vi "App - analyze RUS V6.vi"() -> ()   [LabVIEW 2018] (continued)
              tunnel: w691 -> [_ w703]
              tunnel: w690 -> [_ w702]
              frame False {
                n263 = Initialize Array("" ("name or relative path"), 0 ("dimension size")) -> ()  [unwired: 1 out]
              }
              frame True {
                n264 = call "freq file read-write controller.vi"("Sweep folder path"=w702, "action"=save-read_action."update read list", "save/read"=w703) -> ("save/read OUT"=w701:refnum<vi>)  [unwired: 6 in, 2 out]
                n265 = call "freq file read-write controller.vi"("action"=save-read_action."lookup read number", "Numeric"=w699, "save/read"=w701) -> ("save/read OUT"=w698:refnum<vi>)  [unwired: 6 in, 2 out]
                n266 = call "freq file read-write controller.vi"("action"=save-read_action."copy read from read ring", "save/read"=w698) -> ()  [unwired: 7 in, 3 out]
              }
            }
          }
          frame "new temperature folder" {
            # "input is temperature folder path"
            # "attemp to help to not accidentally \noverwrite existing freqout file NOT FINISHED"
            n267 = call <vilib>:"Check if File or Folder Exists.vi"("path"=w715) -> ("file or folder exists?"=w723:bool, "dup path"=w722:path)  [unwired: 8 in, 1 out]
            n268 = flat-sequence {
              tunnel: w723 -> [w734]
              tunnel: w722 -> [w733]
              tunnel: [w732] -> w716
              tunnel: [w731] -> w721
              tunnel: w713 -> [w730]
              tunnel: w712 -> [w729]
              tunnel: w711 -> [w728]
              tunnel: w710 -> [w727]
              tunnel: w709 -> [w726]
              tunnel: w707 -> [w725]
              tunnel: w720 -> [w802]
              tunnel: w716 -> [w801]
              tunnel: w708 -> [w800]
              frame #0 {
                n269 = case shown="True" w734 {
                  tunnel: w733 -> [_ w754]
                  tunnel: [FALSE w743] -> w732
                  tunnel: [0 w756] -> w731
                  tunnel: w730 -> [_ w748]
                  tunnel: w729 -> [_ w747]
                  tunnel: w728 -> [_ w746]
                  tunnel: w727 -> [_ w745]
                  tunnel: w726 -> [_ w744]
                  tunnel: w725 -> [_ w739]
                  frame False {
                  }
                  frame True {
                    w750 = T40."new"  # action
                    (unwired) FALSE
                    (unwired) TRUE
                    n270 = call "file list from temperatures file V5.vi"("sweep folder path  IN"=w754, "tfolder IN"=w747, "action"=w750, "monotonic segments ON/OFF"=w745) -> ("sweep path array OUT"=w752:T26[], "tfolder OUT"=w749:T30, "OK"=w741:bool, "temperature OUT"=w751:dbl[], "power  OUT"=w738:dbl[], "Magn Field  OUT"=w737:dbl[], "timestamp OUT"=w753:dbl[])  [unwired: 17 in]
                    n271 = And(x=w741, y=FALSE) -> (x .and. y?=w742:bool)
                    n272 = property on="-- loading ..." class="Bool (strict)"("Visible"=w742) -> ()  [unwired: 2 in, 2 out]
                    n273 = property on="-- loading ..." class="Bool (strict)"("Visible"=w744) -> ()  [unwired: 2 in, 2 out]
                    n274 = Array Size(array=w753) -> (size(s)=w756:i32)
                    n275 = Greater Than 0?(x=w756) -> (x > 0?=w743:bool)
                    n276 = case shown="True" w743 {
                      selector: w743 -> [_ w783]
                      tunnel: w753 -> [_ w777]
                      tunnel: w752 -> [_ w759]
                      tunnel: w756 -> [_ w784]
                      tunnel: T27 {"temperature"=0.0, "lorentzian"={"A (VHz)"=0.0, "f (Hz)"=0.0, "G (Hz)"=0.0, "phi(rad)"=0.0, "Q"=0.0, "Norm  Ampl"=0.0, "bg (V)"=0.0+0.0i, "4corners"={"z (-pi/2)"=0.0+0.0i, "z(inf)"=0.0+0.0i, "z (pi/2)"=0.0+0.0i, "z center"=0.0+0.0i, "z(0)"=0.0+0.0i, "radius"=0.0}}, "timestamp(min)"=0.0, "timestamp"=timestamp(0 s since 1904-01-01), "Magn Field(T)"=0.0} ("temperature sweep point") -> [_ w782]
                      tunnel: w751 -> [_ w760]
                      tunnel: w749 -> [_ w775]
                      tunnel: w748 -> [_ w774]
                      tunnel: w746 -> [_ w772]
                      tunnel: w739 -> [_ w767]
                      tunnel: w738 -> [_ w765]
                      tunnel: w737 -> [_ w761]
                      frame False {
                      }
                      frame True {
                        # "set temperature to the middle of the range"
                        n277 = disable-structure shown="Enabled" {
                          disable-tunnel: w777 -> [w797 w799]
                          disable-tunnel: [w796 w799] -> w757
                          frame Enabled {
                            # "set origin to zero"
                            n278 = Array Max & Min(array=w797) -> (min value=w798:dbl)  [unwired: 3 out]
                            n279 = Subtract(x=w797, y=w798) -> (x-y=w796:dbl[])
                          }
                          frame Disabled {
                          }
                        }
                        n280 = local write "in sweep folder"(w783) -> ()
                        n281 = Initialize Array(0.0 ("element"), w784) -> (→"frequency points" →"attenuation points" →"phase points" →"Fit delta f points" →"Fit F points" →"ampl points":dbl[])
                        n282 = Initialize Array(w782, w784) -> (w762:T27[])
                        n283 = Unbundle By Name(w775) -> ("9folder path"=w776:path)
                        n284 = local write "t.folder file path array"(w759) -> ()
                        n285 = local write "tfolder"(w775) -> ()
                        n286 = local write "time points"(w757) -> ()
                        n287 = Array Size(array=w757) -> (size(s)=w787:i32)
                        n288 = local write "9w folder path"(w776) -> ()
                        n289 = Index Array(array=w757, index=0) -> ()  [unwired: 1 out]
                        n290 = Decrement(x=w787) -> (x-1=w788:i32)
                        n291 = Index Array(array=w757, index=w788) -> (element=w768:dbl)
                        n292 = call "cursor window logic V2.vi"("cursor window action"=cursor_window_action."check", "cursor window in"=w774) -> ("cursor window out"=w773:refnum<vi>)  [unwired: 8 in, 1 out]
                        n293 = Threshold 1D Array(2:w768, 3:w757) -> (0:w763:dbl)  [unwired: 1 in]
                        n294 = for {
                          tunnel: w762 -> [w795] mode=indexing
                          tunnel: [w794] -> w758 mode=indexing
                          tunnel: w761 -> [w793] mode=indexing
                          tunnel: w760 -> [w792] mode=indexing
                          tunnel: w759 -> [w791] mode=indexing
                          tunnel: w757 -> [w789] mode=indexing
                          n295 = Unbundle By Name(w791) -> ("last mod"=w790:timestamp)
                          n296 = Bundle By Name(cluster=w795, "temperature"=w792, "Magn Field(T)"=w793, "timestamp(min)"=w789, "timestamp"=w790) -> (w794:T27)
                        }
                        n297 = Index Array(array=w759, index=w763) -> (element=w781:T26)
                        n298 = Unbundle By Name(w781) -> ("temperature"=w780:dbl, "Magn Field(T)"=w764:dbl)
                        n299 = call "cursor window logic V2.vi"("cursor window action"=cursor_window_action."change center", "center"=w768, "cursor window in"=w773) -> ()  [unwired: 7 in, 2 out]
                        n300 = local write "lorentzian points"(w758) -> ()
                        n301 = local write "Magn Field points"(w761) -> ()
                        n302 = local write "temperature points"(w760) -> ()
                        n303 = local write "power points"(w765) -> ()
                        n304 = local write "temperature(K)"(w780) -> ()
                        n305 = local write "magn field(T)"(w764) -> ()
                        n306 = local write "time (min)"(w768) -> ()
                        n307 = local write "current index"(w763) -> ()
                        n308 = call "replace cursor - plot ref.vi"("action"=enum16{"", "read", "write"}."write", "cursor index"=0, "new X"=w768, "Plot ref in"=w772) -> ()  [unwired: 5 in, 3 out]
                        n309 = call "follow the peak controller.vi"("action"=follow_the_peak_action."make dirty", "follow the peak ref"=w767) -> ()  [unwired: 8 in, 2 out]
                      }
                    }
                  }
                }
              }
              frame #1 {
                n310 = case shown="True" w801 {
                  tunnel: w802 -> [_ w806]
                  tunnel: w800 -> [_ w805]
                  frame False {
                  }
                  frame True {
                    w807 = "new temperature"  # t.folder
                    n311 = Generate User Event(user event=w806, event data cluster=w807) -> (error out=w803:errorcluster)  [unwired: 2 in, 1 out]
                    n312 = Generate User Event(user event=w805, event data cluster="redraw:time" ("t.folder"), error in=w803) -> ()  [unwired: 1 in, 2 out]
                  }
                }
              }
            }
            n313 = call "freq file read-write controller.vi"("action"=save-read_action."init save file", "save/read"=w706) -> ()  [unwired: 7 in, 3 out]
            n314 = Select(t=u32 16777222, s=w716, f=u32 16719872) -> (s? t:f=w717:u32)
            n315 = property on="Sweep folder path" class="Path"("Text.TextColor"=w717) -> ()  [unwired: 2 in, 2 out]
            n316 = case shown="True" w716 {
              tunnel: T37."Enabled" ("Disabled") -> [_ w724]
              frame False {
              }
              frame True {
                n317 = property on="Tab : temperature folder" class="TabCtl (strict)"("DisabledEnum"=w724) -> ()  [unwired: 2 in, 2 out]
              }
            }
            "files in t.folder" <- w721
          }
          frame "not in temperature folder" {
            w808 = TRUE  # Visible
            w809 = T37."Disabled and Grayed Out"  # Disabled
            n318 = local write "in sweep folder"(w810) -> ()
            n319 = property on="back to temperature folder" class="Bool"("Visible"=w808) -> ()  [unwired: 2 in, 2 out]
            n320 = property on="Tab : temperature folder" class="TabCtl (strict)"("DisabledEnum"=w809) -> ()  [unwired: 2 in, 2 out]
          }
          frame "update freq/atten" {
            n321 = case shown="True" w813 {
              tunnel: w821 -> [_ w831]
              tunnel: w820 -> [_ w830]
              tunnel: w819 -> [_ w829]
              tunnel: w818 -> [_ w828]
              tunnel: w817 -> [_ w827]
              tunnel: w816 -> [_ w826]
              tunnel: w815 -> [_ w825]
              tunnel: w814 -> [_ w824]
              tunnel: w812 -> [_ w823]
              tunnel: w811 -> [_ w822]
              frame False {
              }
              frame True {
                n322 = flat-sequence {
                  tunnel: w831 -> [_]
                  tunnel: w829 -> [w868]
                  tunnel: w828 -> [w867]
                  tunnel: w827 -> [w866]
                  tunnel: w826 -> [w865]
                  tunnel: w825 -> [w864]
                  tunnel: w824 -> [w837]
                  tunnel: w823 -> [w836]
                  tunnel: w822 -> [w834]
                  tunnel: w830 -> [w875]
                  frame #0 {
                    w841 = enum16{"", "read", "write"}."write"  # action
                    w845 = enum16{"", "read", "write"}."write"  # action
                    n323 = local read "time (min)"() -> (w854:dbl)
                    n324 = Threshold 1D Array(2:w854, 3:w867) -> (0:w833:dbl)  [unwired: 1 in]
                    n325 = Index Array(array=w866, index=w833) -> (element=w847:dbl)
                    n326 = Index Array(array=w834, index=w833) -> (element=w832:dbl)
                    n327 = local read "attenuation points"() -> (w859:dbl[])
                    n328 = local read "frequency points"() -> (w860:dbl[])
                    n329 = call "freq file read-write controller.vi"("action"=save-read_action."saved file dirty", "save/read"=w836) -> ()  [unwired: 7 in, 3 out]
                    n330 = in-place {
                      in-place-border: w868 -> [w871]
                      in-place-border: w847 -> [w870]
                      in-place-border: w832 -> [w869]
                      n331 = in-place-array #1(w865, w833) -> (w873:T27)
                      n332 = Bundle By Name(cluster=w873, "lorentzian"=w871, "temperature"=w870, "Magn Field(T)"=w869) -> (w872:T27)
                      n333 = in-place-array #1(w872) -> (w855:T27[])  [unwired: 1 out]
                    }
                    n334 = Unbundle By Name(w868) -> ("A (VHz)"=w853:dbl, "phi(rad)"=w857:dbl, "G (Hz)"=w861:dbl, "f (Hz)"=w843:dbl)
                    n335 = local read "phase points"() -> (w858:dbl[])
                    n336 = local read "ampl points"() -> (w852:dbl[])
                    n337 = Replace Array Subset(array=w858, new element=w857, index=w833) -> (w856:dbl[])
                    n338 = Replace Array Subset(array=w852, new element=w853, index=w833) -> (w851:dbl[])
                    n339 = Replace Array Subset(array=w859, new element=w861, index=w833) -> (w862:dbl[])
                    n340 = Replace Array Subset(array=w860, new element=w843, index=w833) -> (w863:dbl[])
                    n341 = Build Array(w847) -> (w848:dbl[])
                    n342 = local write "lorentzian points"(w855) -> ()
                    n343 = local write "phase points"(w856) -> ()
                    n344 = local write "frequency points"(w863) -> ()
                    n345 = local write "attenuation points"(w862) -> ()
                    n346 = local write "ampl points"(w851) -> ()
                    n347 = call "fit function selector.vi"("fit using"=w837, "temperature"=w848, "best fit parameters"=w864) -> ("freq out"=w849:dbl[])  [unwired: 6 in, 2 out]
                    n348 = Index Array(array=w849, index=0 ("cursor index")) -> (element=w842:dbl)
                    n349 = Subtract(x=w843, y=w842) -> (x-y=w839:dbl)
                    n350 = control-ref of="Plot: frequency vs T"() -> (w846:refnum<vi>)
                    n351 = call "replace cursor - plot ref.vi"("action"=w845, "cursor index"=1, "new  Y"=w843, "Plot ref in"=w846) -> ()  [unwired: 5 in, 3 out]
                    n352 = control-ref of="Plot: delta f"() -> (w838:refnum<vi>)
                    n353 = call "replace cursor - plot ref.vi"("action"=w841, "cursor index"=1, "new  Y"=w839, "Plot ref in"=w838) -> ()  [unwired: 5 in, 3 out]
                  }
                  frame #1 {
                    w874 = "calculation finished"  # talk to the first loop
                    n354 = Generate User Event(user event=w875, event data cluster=w874) -> ()  [unwired: 2 in, 2 out]
                  }
                }
              }
            }
          }
          frame "clear freq points" {
            n355 = case shown="True" w877 {
              tunnel: w879 -> [_ w884]
              tunnel: w878 -> [_ w883]
              tunnel: w876 -> [_ w880]
              frame False {
              }
              frame True {
                n356 = local read "attenuation points"() -> (w896:dbl[])
                n357 = local read "frequency points"() -> (w897:dbl[])
                n358 = local read "Fit delta f points"() -> (w890:dbl[])
                n359 = local read "phase points"() -> (w886:dbl[])
                n360 = local read "ampl points"() -> (w882:dbl[])
                n361 = local read "Fit F points"() -> (w889:dbl[])
                n362 = Unbundle By Name(T27 {"temperature"=0.0, "lorentzian"={"A (VHz)"=0.0, "f (Hz)"=0.0, "G (Hz)"=0.0, "phi(rad)"=0.0, "Q"=0.0, "Norm  Ampl"=0.0, "bg (V)"=0.0+0.0i, "4corners"={"z (-pi/2)"=0.0+0.0i, "z(inf)"=0.0+0.0i, "z (pi/2)"=0.0+0.0i, "z center"=0.0+0.0i, "z(0)"=0.0+0.0i, "radius"=0.0}}, "timestamp(min)"=0.0, "timestamp"=timestamp(0 s since 1904-01-01), "Magn Field(T)"=0.0} ("temperature sweep point")) -> ("lorentzian"=w894:T11)
                n363 = for {
                  shift-right: [w913] -> w892
                  shift-left: w896 -> [w915]
                  shift-right: [w906] -> w893
                  shift-left: w883 -> [w903]
                  shift-right: [w914] -> w891
                  shift-left: w897 -> [w916]
                  tunnel: w884 -> [w904] mode=indexing
                  tunnel: w894 -> [w905]
                  shift-right: [w912] -> w888
                  shift-left: w890 -> [w909]
                  shift-right: [w911] -> w887
                  shift-left: w889 -> [w910]
                  shift-right: [w907] -> w885
                  shift-left: w886 -> [w908]
                  shift-right: [w899] -> w881
                  shift-left: w882 -> [w900]
                  tunnel: w880 -> [w898] mode=indexing
                  i -> [w902]
                  w901 = 0.0 ("new element/subarray")
                  n364 = in-place {
                    in-place-border: w905 -> [w921]
                    in-place-border: w904 -> [w920]
                    in-place-border: w898 -> [w917]
                    n365 = in-place-array #2(w903, w902) -> (w918:T27)
                    n366 = Bundle By Name(cluster=w918, "Magn Field(T)"=w917, "temperature"=w920, "lorentzian"=w921) -> (w919:T27)
                    n367 = in-place-array #2(w919) -> (w906:T27[])  [unwired: 1 out]
                  }
                  n368 = Replace Array Subset(array=w916, new element=w901, index=w902) -> (w914:dbl[])
                  n369 = Replace Array Subset(array=w909, new element=w901, index=w902) -> (w912:dbl[])
                  n370 = Replace Array Subset(array=w910, new element=w901, index=w902) -> (w911:dbl[])
                  n371 = Replace Array Subset(array=w900, new element=w901, index=w902) -> (w899:dbl[])
                  n372 = Replace Array Subset(array=w908, new element=w901, index=w902) -> (w907:dbl[])
                  n373 = Replace Array Subset(array=w915, new element=w901, index=w902) -> (w913:dbl[])
                }
                n374 = local write "lorentzian points"(w893) -> ()
                n375 = local write "frequency points"(w891) -> ()
                n376 = local write "attenuation points"(w892) -> ()
                n377 = local write "phase points"(w885) -> ()
                n378 = local write "Fit delta f points"(w888) -> ()
                n379 = local write "Fit F points"(w887) -> ()
                n380 = local write "ampl points"(w881) -> ()
              }
            }
          }
          frame "new temperature" {
            n381 = case shown="True" w923 {
              tunnel: w930 -> [_ w941]
              tunnel: w923 -> [_ w940]
              tunnel: w929 -> [_ w939]
              tunnel: w928 -> [_ w938]
              tunnel: w927 -> [_ w937]
              tunnel: w926 -> [_ w936]
              tunnel: w925 -> [_ w935]
              tunnel: w924 -> [_ w934]
              tunnel: w922 -> [_ w931]
              frame False {
              }
              frame True {
                # "calculation  for the next temperature uses the two cursor brackets that are set here"
                # "logic : this and othe othe events are chaned:\n any of them induce the down stream events to execute"
                n382 = flat-sequence {
                  tunnel: w940 -> [w967]
                  tunnel: w939 -> [w964]
                  tunnel: w938 -> [w956]
                  tunnel: w937 -> [w957]
                  tunnel: w936 -> [w963]
                  tunnel: w935 -> [w962]
                  tunnel: [w961] -> w943
                  tunnel: [w960] -> w942
                  tunnel: w931 -> [w948]
                  tunnel: w934 -> [w988]
                  tunnel: w943 -> [w987]
                  tunnel: w942 -> [w979]
                  tunnel: w933 -> [w982]
                  tunnel: w932 -> [w980]
                  tunnel: w941 -> [w990]
                  frame #0 {
                    n383 = Unbundle By Name(w962) -> ("G (Hz)"=w953:dbl, "f (Hz)"=w958:dbl)
                    n384 = call "follow the peak controller.vi"("action"=follow_the_peak_action."check", "follow the peak ref"=w948) -> ("follow the peak OUT"=w945:T7)  [unwired: 8 in, 1 out]
                    n385 = local read "time (min)"() -> (w961:dbl)
                    n386 = Unbundle By Name(w945) -> ("omega ?"=w947:bool)
                    n387 = Threshold 1D Array(2:w961, 3:w963) -> (0:w966:dbl)  [unwired: 1 in]
                    n388 = Compound Arithmetic op=AND(w967, w947) -> (w954:bool)
                    n389 = case shown="True" w954 {
                      tunnel: w958 -> [_ w977]
                      tunnel: w957 -> [_ w976]
                      tunnel: w956 -> [_ w975]
                      tunnel: [w968 FALSE] -> _
                      tunnel: [w968 w973] -> w955
                      tunnel: w953 -> [_ w971]
                      tunnel: w945 -> [_ w969]
                      frame False {
                        w968 = FALSE
                      }
                      frame True {
                        n390 = call "follow the peak.vi"("omega(0)"=w977, "gamma"=w971, "follow the peak Con"=w969, "cursor bracket - data 2"=w975, "cursor bracket - fragment 2"=w976) -> ("interpolated omega"=→"interpolated omega":dbl, "interpolated gamma"=→"interpolated gamma":dbl, "follow the peak is clean out"=w973:bool)  [unwired: 8 in]
                      }
                    }
                    n391 = Index Array(array=w964, index=w966) -> (element=w965:T26)
                    n392 = Unbundle By Name(w965) -> ("temperature"=w960:dbl, "file path"=w959:path, "Magn Field(T)"=w944:dbl)
                    n393 = Compound Arithmetic op=AND(w955, w954) -> (w952:bool)
                    n394 = Select(t=follow_the_peak_action."make clean" ("action"), s=w952, f=follow_the_peak_action."make clean" ("action")) -> (s? t:f=w949:T33)
                    n395 = local write "temperature(K)"(w960) -> ()
                    n396 = local write "magn field(T)"(w944) -> ()
                    n397 = local write "file path"(w959) -> ()
                    n398 = call "follow the peak controller.vi"("action"=w949, "follow the peak ref"=w948) -> ()  [unwired: 8 in, 2 out]
                  }
                  frame #1 {
                    w981 = enum16{"", "read", "write"}."write"  # action
                    w984 = enum16{"", "read", "write"}."write"  # action
                    w986 = enum16{"", "read", "write"}."write"  # action
                    n399 = call "replace cursor - plot ref.vi"("action"=w984, "cursor index"=1, "new X"=w979, "Plot ref in"=w982) -> ()  [unwired: 5 in, 3 out]
                    n400 = call "replace cursor - plot ref.vi"("action"=w981, "cursor index"=1, "new X"=w979, "Plot ref in"=w980) -> ()  [unwired: 5 in, 3 out]
                    n401 = call "replace cursor - plot ref.vi"("action"=w986, "cursor index"=5, "new  Y"=w979, "new X"=w987, "Plot ref in"=w988) -> ()  [unwired: 4 in, 3 out]
                  }
                  frame #2 {
                    # "send \"new file\" event"
                    n402 = Generate User Event(user event=w990, event data cluster="calc:new file" ("event data")) -> ()  [unwired: 2 in, 2 out]
                  }
                }
                n403 = control-ref of="Plot: frequency vs T"() -> (w933:refnum<vi>)
                n404 = control-ref of="Plot: delta f"() -> (w932:refnum<vi>)
              }
            }
          }
          frame "set time to left" {
            # "cursor bracket -- bounds"
            n405 = call "cursor window logic V2.vi"("cursor window action"=cursor_window_action."check", "cursor window in"=w1002) -> ("cursor window out"=w1001:T24)  [unwired: 8 in, 1 out]
            n406 = Unbundle By Name(w1001) -> ("left"=w1000:dbl)
            n407 = Threshold 1D Array(2:w1000, 3:w998) -> (0:w992:dbl)  [unwired: 1 in]
            n408 = Index Array(array=w999, index=w992) -> (element=w996:dbl)
            n409 = Index Array(array=w993, index=w992) -> (element=w991:dbl)
            n410 = Index Array(array=w998, index=w992) -> (element=w997:dbl)
            n411 = local write "temperature(K)"(w996) -> ()
            n412 = local write "magn field(T)"(w991) -> ()
            n413 = local write "time (min)"(w997) -> ()
            n414 = Generate User Event(user event=w994, event data cluster="new temperature" ("event data")) -> ()  [unwired: 2 in, 2 out]
          }
          frame "follow the peak -- init" {
            n415 = call "follow the peak controller.vi"("action"=follow_the_peak_action."make dirty", "follow the peak ref"=w1005) -> ()  [unwired: 8 in, 2 out]
          }
          frame "next peak" {
            # "\";\""
            n416 = Unbundle By Name(w1012) -> ("f (Hz)"=w1007:dbl)
            n417 = call "freq file read-write controller.vi"("action"=save-read_action."nearest right", "Numeric"=w1007, "save/read"=w1009) -> ("Numeric out"=w1006:dbl)  [unwired: 6 in, 2 out]
            n418 = call "Q - not nan and gtr than zero.vi"("Numeric"=w1006) -> ("Boolean"=w1013:bool)  [unwired: 10 in]
            n419 = case shown="True" w1013 {
              tunnel: w1011 -> [_ w1016]
              tunnel: w1006 -> [_ w1015]
              tunnel: w1010 -> [_ w1014]
              frame False {
              }
              frame True {
                n420 = flat-sequence {
                  tunnel: w1016 -> [w1019]
                  tunnel: w1015 -> [w1018]
                  tunnel: w1014 -> [w1020]
                  frame #0 {
                    n421 = call "cursor window logic V2.vi"("cursor window action"=cursor_window_action."change center", "center"=w1018, "cursor window in"=w1019) -> ()  [unwired: 7 in, 2 out]
                  }
                  frame #1 {
                    w1021 = "calc:new cursor bracket"  # event data
                    n422 = Generate User Event(user event=w1020, event data cluster=w1021) -> ()  [unwired: 2 in, 2 out]
                  }
                }
              }
            }
          }
          frame "increment peak index" {
            # ":"
            n423 = call "freq file read-write controller.vi"("action"=save-read_action."increment read from", "save/read"=w1023) -> ()  [unwired: 7 in, 3 out]
          }
          frame "latest temperature" {
            w1034 = enum16{"hide", "show x", "show y", "show (x,y)"}."hide"  # label
            w1035 = enum16{"", "read", "write"}."write"  # action
            w1036 = "same"  # next temperature
            n424 = Array Size(array=w1033) -> (size(s)=w1037:i32)
            n425 = Decrement(x=w1037) -> (x-1=w1025:i32)
            n426 = Index Array(array=w1032, index=w1025) -> (element=w1031:dbl)
            n427 = Index Array(array=w1026, index=w1025) -> (element=w1024:dbl)
            n428 = Index Array(array=w1033, index=w1025) -> (element=w1027:dbl)
            n429 = local write "magn field(T)"(w1024) -> ()
            n430 = local write "time (min)"(w1027) -> ()
            n431 = local write "temperature(K)"(w1031) -> ()
            n432 = call "replace cursor - plot ref.vi"("label"=w1034, "action"=w1035, "cursor index"=0, "new X"=w1027, "Plot ref in"=w1029) -> ()  [unwired: 4 in, 3 out]
            n433 = Generate User Event(user event=w1028, event data cluster=w1036) -> ()  [unwired: 2 in, 2 out]
          }
        }
      }
      event "Sweep folder path": Value Change; "Sweep folder path": Mouse Down {
        n434 = event-data() -> ()  [unwired: 1 in, 1 out]
        n435 = flat-sequence {
          tunnel: w1040 -> [w1043]
          tunnel: [w1042] -> w1039
          tunnel: [w1045] -> _
          tunnel: w1039 -> [w1046]
          tunnel: w1038 -> [w1047]
          frame #0 {
            w1044 = "new temperature folder"  # t.folder
            n436 = Generate User Event(user event=w1043, event data cluster=w1044) -> (error out=w1042:errorcluster)  [unwired: 2 in, 1 out]
          }
          frame #1 {
            n437 = Generate User Event(user event=w1047, event data cluster="redraw:time", error in=w1046) -> (error out=w1045:errorcluster)  [unwired: 1 in, 1 out]
          }
        }
      }
      event "back to temperature folder": Value Change {
        w1049 = FALSE  # Visible
        w1050 = T37."Enabled"  # Disabled
        n438 = event-data() -> ()  [unwired: 1 in, 2 out]
        n439 = property on="Tab : temperature folder" class="TabCtl (strict)"("DisabledEnum"=w1050) -> ()  [unwired: 2 in, 2 out]
        n440 = property on="back to temperature folder" class="Bool"("Visible"=w1049) -> ()  [unwired: 2 in, 2 out]
      }
      event Value Change {
        w1057 = "update delta freq"  # t.folder
        w1060 = "read freq file"  # t.folder
        n441 = event-data() -> ()  [unwired: 1 in, 1 out]
        n442 = case shown="False" w1054 {
          tunnel: w1059 -> [w1061 w1063]
          tunnel: [w1061 w1062] -> w1058
          frame False {
          }
          frame True {
            w1064 = "clear freq points"  # t.folder
            n443 = Generate User Event(user event=w1063, event data cluster=w1064) -> (user event out=w1062:refnum<user-event>)  [unwired: 2 in, 1 out]
          }
        }
        n444 = call "freq file read-write controller.vi"("action"=save-read_action."read event", "save/read"=w1053) -> ()  [unwired: 7 in, 3 out]
        n445 = Generate User Event(user event=w1058, event data cluster=w1060) -> (user event out=w1055:refnum<user-event>, error out=w1056:errorcluster)  [unwired: 2 in]
        n446 = Generate User Event(user event=w1055, event data cluster=w1057, error in=w1056) -> ()  [unwired: 1 in, 2 out]
      }
      event Value Change {
        w1067 = "clear freq points"  # t.folder
        n447 = event-data() -> ()  [unwired: 1 in, 1 out]
        n448 = call "freq file read-write controller.vi"("action"=save-read_action."erase event", "save/read"=w1065) -> ()  [unwired: 7 in, 3 out]
        n449 = Generate User Event(user event=w1068, event data cluster=w1067) -> ()  [unwired: 2 in, 2 out]
      }
      event Value Change {
        w1071 = "write freq file"  # t.folder
        n450 = event-data() -> ()  [unwired: 1 in, 1 out]
        n451 = call "freq file read-write controller.vi"("action"=save-read_action."read event", "save/read"=w1069) -> ()  [unwired: 7 in, 3 out]
        n452 = Generate User Event(user event=w1072, event data cluster=w1071) -> ()  [unwired: 2 in, 2 out]
      }
      event Value Change; Mouse Enter {
        n453 = event-data() -> ()  [unwired: 1 in, 3 out]
      }
      event "file path": Value Change; "file path": Mouse Down {
        w1080 = "not in temperature folder"  # t.folder
        n454 = event-data() -> ()  [unwired: 1 in, 1 out]
        n455 = local read "file path"() -> (w1073:path)
        n456 = call <vilib>:"Check if File or Folder Exists.vi"("path"=w1073) -> ("file or folder exists?"=w1075:bool)  [unwired: 8 in, 2 out]
        n457 = Generate User Event(user event=w1081, event data cluster=w1080) -> (error out=w1079:errorcluster)  [unwired: 2 in, 1 out]
        n458 = Select(t=u32 16777222, s=w1075, f=u32 16719872) -> (s? t:f=w1076:u32)
        n459 = property on="file path" class="Path"("Text.TextColor"=w1076) -> ()  [unwired: 2 in, 2 out]
        n460 = case shown="True" w1075 {
          tunnel: w1074 -> [_ w1084]
          tunnel: w1079 -> [_ w1083]
          frame False {
          }
          frame True {
            w1082 = "calc:new file"  # calc
            n461 = Generate User Event(user event=w1084, event data cluster=w1082, error in=w1083) -> ()  [unwired: 1 in, 2 out]
          }
        }
      }
      event Timeout {
        n462 = event-data() -> ()  [unwired: 1 in, 2 out]
      }
    }
  }
  n463 = Create User Event(user event datatype=w30) -> (user event=w43:refnum<user-event>)  [unwired: 1 in, 1 out]
  n464 = Create User Event(user event datatype=w46) -> (user event=w45:refnum<user-event>)  [unwired: 1 in, 1 out]
  n465 = Create User Event(user event datatype=w40) -> (user event=w39:refnum<user-event>)  [unwired: 1 in, 1 out]
  n466 = Create User Event(user event datatype=w31) -> (user event=w27:refnum<user-event>)  [unwired: 1 in, 1 out]
  n467 = Create User Event(user event datatype=w38) -> (user event=w37:refnum<user-event>)  [unwired: 1 in, 1 out]
  n468 = call "cursor window - init all.vi"("cursor bracket:  Time 2"=w22, "cursor bracket: fragment 2"=w25, "cursor bracket:  All, zoom 2"=w23, "cursor bracket:  All, data window 2"=w24, "Plot: Time"=w21, "Plot:  Fragment"=w26, "cursor bracket:  All, show 2"=w19, "Plot: All"=w20) -> ()
  n469 = control-ref of="slide control"() -> (w4:refnum<vi>)
  n470 = register-events(w17, w44, w43, w45, w39, w27, w37, w33) -> (reference out=w49:refnum<event-registration>)  [unwired: 2 in, 1 out]
  n471 = call "slide controller.vi"("slide action"=slide_action."init", "slide control"=w4) -> ("slide control OUT"=w3:refnum<vi>)  [unwired: 6 in, 3 out]
  n472 = while {
    tunnel: w49 -> [w1133]
    tunnel: w16 -> [w1132]
    tunnel: w17 -> [w1131]
    tunnel: w44 -> [w1129]
    tunnel: w45 -> [w1127]
    tunnel: w43 -> [w1126]
    tunnel: w39 -> [w1125]
    tunnel: w27 -> [w1124]
    tunnel: w18 -> [w1123]
    tunnel: w37 -> [w1122]
    tunnel: w28 -> [_]
    tunnel: w20 -> [_]
    tunnel: w3 -> [_]
    i -> [w1093]
    stop <- FALSE ("Boolean") stop-if-true
    n473 = local read "cursor bracket: All, data window"() -> (w1103:T24)
    n474 = local read "parameters: center detection"() -> (w1116:T21)
    n475 = Wait (ms)(milliseconds to wait=u32 3) -> ()  [unwired: 1 out]
    n476 = Equal To 0?(x=w1093) -> (x = 0?=w1092:bool)
    n477 = local read "parameters: wavepacket"() -> (w1113:T16)
    n478 = local read "cursor bracket: fragment"() -> (w1104:T24)
    n479 = local read "parameters: omega map"() -> (w1115:T22)
    n480 = control-ref of="save/read"() -> (w1089:refnum<vi>)
    n481 = local read "plot scale: Geometry"() -> (w1121:T28)
    n482 = local read "cursor bracket: Time"() -> (w1101:T24)
    n483 = local read "Sweep folder path"() -> (w1112:path)
    n484 = local read "in sweep folder"() -> (w1118:bool)
    n485 = local read "complex region"() -> (w1114:T25)
    n486 = local read "9w folder path"() -> (w1111:path)
    n487 = control-ref of="follow the peak"() -> (w1091:refnum<vi>)
    n488 = local read "lorentzian"() -> (w1117:T11)
    n489 = control-ref of="Plot: All"() -> (w1102:refnum<vi>)
    n490 = control-ref of="Plot: complex plane"() -> (w1105:refnum<vi>)
    n491 = control-ref of="Plot: fragment"() -> (w1106:refnum<vi>)
    n492 = control-ref of="Plot: Time"() -> (w1100:refnum<vi>)
    n493 = control-ref of="slide control"() -> (w1090:refnum<vi>)
    n494 = local read "section"() -> (w1119:i32)
    n495 = local read "tfolder"() -> (w1120:T30)
    n496 = control-ref of="cursor bracket: All, data window"() -> (w1108:refnum<vi>)
    n497 = control-ref of="cursor bracket: All,  zoom"() -> (w1109:refnum<vi>)
    n498 = control-ref of="cursor bracket: fragment"() -> (w1107:refnum<vi>)
    n499 = control-ref of="cursor bracket: Time"() -> (w1110:refnum<vi>)
    n500 = control-ref of="Plot: frequency vs H"() -> (w1086:refnum<vi>)
    n501 = control-ref of="Plot: attenuation vs H"() -> (w1085:refnum<vi>)
    n502 = control-ref of="Plot: gamma vs power"() -> (w1087:refnum<vi>)
    n503 = control-ref of="Plot: frequency vs power"() -> (w1088:refnum<vi>)
    n504 = control-ref of="Plot: Time"() -> (w1094:refnum<vi>)
    n505 = control-ref of="Plot: frequency vs T"() -> (w1097:refnum<vi>)
    n506 = control-ref of="Plot: attenuation vs T"() -> (w1098:refnum<vi>)
    n507 = control-ref of="Plot: df/dT"() -> (w1099:refnum<vi>)
    n508 = control-ref of="Plot: delta f"() -> (w1096:refnum<vi>)
    n509 = event shown="[18] <redraw>: User Event" {
      selector: w1133 -> [_ _ _ _ _ _ _ _ _ _ _ _ _ _ _ _ _ _ _ _ _ _ _ _ _ _ _ _ _ _ _ _ _ _ _ _ _ _ _ _ _ _ _ _ _]
      dyn-events: _ -> [_ _ _ _ _ _ _ _ _ _ _ _ _ _ _ _ _ _ _ _ _ _ _ _ _ _ _ _ _ _ _ _ _ _ _ _ _ _ _ _ _ _ _ _ _]
      timeout: _ -> [_ _ _ _ _ _ _ _ _ _ _ _ _ _ _ _ _ _ _ _ _ _ _ _ _ _ _ _ _ _ _ _ _ _ _ _ _ _ _ _ _ _ _ _ _]
      tunnel: w1132 -> [_ _ w1213 _ _ _ _ w1577 _ _ _ _ _ _ _ _ _ _ _ _ _ _ _ _ _ _ _ _ _ _ _ _ _ _ _ _ _ _ _ _ _ _ w2370 w2385 w2415]
      tunnel: w1131 -> [w1142 _ w1221 _ _ _ _ w1576 _ _ _ _ _ _ _ w1664 _ _ w1827 _ _ _ _ _ _ _ _ _ _ _ _ _ _ _ w2284 _ _ _ _ _ w2364 w2367 _ _ _]
      tunnel: [_ _ _ _ _ _ _ _ _ _ _ _ _ _ _ _ _ _ _ _ _ _ _ _ _ _ _ _ _ _ _ _ _ _ _ "help (h)" _ _ _ _ "plot filter progress?" _ _ _ _] -> _
      tunnel: [_ _ _ _ _ w1555 _ _ _ _ _ _ _ _ _ _ _ _ _ _ _ _ _ _ _ _ _ _ _ _ _ _ _ _ _ "help toggle" _ _ _ _ _ _ _ _ _] -> _
      tunnel: FALSE ("Boolean") -> [_ _ _ _ _ w1555 w1562 _ _ _ _ _ _ _ _ _ _ _ _ _ _ _ _ _ _ _ _ _ _ _ _ _ _ _ _ _ _ _ _ _ _ _ w2369 _ _]
      tunnel: w1129 -> [_ w1203 w1222 _ _ w1557 w1565 _ _ _ _ w1611 _ _ _ w1665 _ _ _ _ _ _ _ _ _ _ _ _ _ _ _ _ _ _ _ _ _ _ _ _ _ _ _ _ _]
      tunnel: TRUE ("Boolean") -> [_ _ _ _ _ w1556 _ _ _ _ _ _ _ _ _ _ _ _ _ _ _ _ _ _ _ _ _ _ _ _ _ _ _ _ _ _ _ _ _ _ _ _ _ _ _]
      tunnel: [_ _ _ _ _ _ w1563 _ w1599 w1603 w1606 w1609 _ _ _ _ _ _ _ _ _ _ _ _ _ _ _ _ _ _ _ _ _ _ _ _ _ _ _ _ _ _ _ _ _] -> _
      tunnel: [_ _ _ _ _ _ _ _ _ "c.plane scale" _ _ _ _ _ _ _ _ _ _ _ _ _ _ _ _ _ _ _ _ _ _ _ _ _ _ _ _ _ _ _ _ _ _ _] -> _
      tunnel: w1127 -> [_ _ w1220 _ _ _ _ _ _ _ _ _ _ _ _ _ _ _ _ _ _ _ _ _ _ _ _ _ _ _ _ _ _ _ _ _ _ _ _ _ _ _ _ _ _]
      tunnel: [_ _ _ _ _ _ _ _ _ _ "show all cursors (c)" _ _ _ _ _ _ _ _ _ _ _ _ _ _ _ _ _ _ _ _ _ _ _ _ _ _ _ _ _ _ _ _ _ _] -> _
      tunnel: w1126 -> [_ _ w1215 _ _ _ _ w1572 _ _ w1607 _ _ _ _ _ _ _ _ _ _ _ _ _ _ _ _ _ _ _ _ _ _ _ _ _ _ _ _ _ _ _ _ _ _]
      tunnel: [_ _ _ _ _ _ w1562 _ _ _ _ _ "show all pallets (p)" _ _ _ _ _ _ _ _ _ _ _ _ _ _ _ _ _ _ _ _ _ _ _ _ _ _ _ _ _ _ _ _] -> _
      tunnel: w1125 -> [_ _ w1219 _ _ _ _ _ _ _ _ _ w1614 _ _ _ _ _ _ _ _ _ _ _ _ _ _ _ _ _ _ _ _ _ _ _ _ _ _ _ _ _ _ _ _]
      tunnel: [_ _ _ _ _ _ _ w1571 _ _ _ _ w1612 _ _ _ _ _ _ _ _ _ _ _ _ _ _ _ _ _ _ _ _ _ _ _ _ _ _ _ _ _ _ _ _] -> _
      tunnel: w1124 -> [_ _ w1218 _ _ _ _ w1573 _ w1602 _ _ _ _ _ w1663 _ _ w1797 _ w2141 _ _ _ _ _ _ _ _ _ _ _ _ _ _ _ _ _ _ _ _ _ _ _ _]
      tunnel: w1123 -> [w1141 _ w1217 w1432 w1486 _ _ w1575 _ _ _ _ _ _ _ _ _ _ _ _ _ _ w2160 _ _ _ _ _ _ _ _ _ _ _ _ _ _ _ _ _ _ _ _ _ _]
      tunnel: w1122 -> [_ _ w1216 _ _ _ _ _ _ _ _ _ _ _ _ _ _ _ _ _ _ _ _ _ _ _ _ _ _ _ _ _ _ _ _ _ _ _ _ _ _ _ _ _ _]
      tunnel: w1121 -> [_ _ _ _ _ _ _ _ _ _ _ _ _ _ _ _ _ _ _ _ _ _ _ _ _ _ _ _ _ _ _ _ _ _ _ _ _ _ _ _ _ _ _ _ _]
      tunnel: [_ _ _ _ _ _ _ _ _ _ _ _ _ _ _ _ _ _ _ _ _ _ _ _ _ _ _ _ _ _ w2250 _ _ _ _ _ _ _ _ _ _ _ _ _ _] -> _
      tunnel: w1120 -> [_ _ _ _ _ _ _ _ _ _ _ _ _ _ _ _ _ _ w1817 _ _ _ _ _ _ _ _ _ _ _ _ _ _ w2276 w2287 _ _ _ _ _ _ _ _ _ _]
      tunnel: w1119 -> [_ _ _ _ _ _ _ _ _ _ _ _ _ _ _ _ _ _ _ _ _ _ _ _ _ _ _ _ _ _ _ _ _ _ w2286 _ _ _ _ _ _ _ _ _ _]
      tunnel: w1118 -> [_ _ w1209 _ w1481 _ _ _ _ _ _ _ _ _ _ _ _ _ w1814 _ _ _ _ _ _ _ _ _ _ _ _ _ _ _ _ _ _ _ _ _ _ _ _ _ _]
      tunnel: w1117 -> [_ _ w1210 w1430 _ _ _ _ _ _ _ _ _ _ _ w1662 w1715 _ w1819 _ _ _ w2162 _ w2184 _ _ _ w2232 w2241 _ _ _ _ _ _ _ _ _ _ _ _ _ _ _]
      tunnel: w1116 -> [w1140 _ _ w1428 _ _ _ _ _ _ _ _ _ _ _ _ w1714 _ w1818 _ _ _ _ _ _ _ _ _ _ _ _ _ _ _ _ _ _ _ _ _ _ _ _ _ _]
      tunnel: w1115 -> [_ _ _ w1429 _ _ _ _ _ _ _ _ _ _ _ _ _ _ w1816 _ _ _ _ _ _ _ _ _ _ _ _ _ _ _ _ _ _ _ _ _ _ _ _ _ _]
      tunnel: w1114 -> [_ _ _ _ _ _ _ _ _ _ _ _ _ _ _ _ w1713 _ w1813 _ _ _ _ _ _ _ _ _ _ _ _ _ _ _ _ _ _ _ _ _ _ _ _ _ _]
      tunnel: w1113 -> [_ _ _ _ _ _ _ _ _ _ _ _ _ _ _ _ _ _ w1815 _ _ _ _ _ _ _ _ _ _ _ _ _ _ _ _ _ _ _ _ _ _ _ _ _ _]
      tunnel: w1112 -> [_ _ w1207 _ _ _ _ _ _ _ _ _ _ _ _ _ _ _ _ _ _ _ _ _ _ _ _ _ _ _ _ _ _ _ _ _ _ _ _ _ _ _ _ _ _]
      tunnel: w1111 -> [_ _ _ _ _ _ _ _ _ _ _ _ _ _ _ _ _ _ _ _ _ _ w2164 _ _ _ _ _ _ _ _ _ _ _ _ _ _ _ _ _ _ _ _ _ _]
      tunnel: w1110 -> [_ _ _ _ _ _ _ _ _ _ _ _ _ _ _ _ _ _ _ _ _ w2144 _ _ _ _ _ _ _ _ _ _ _ _ _ _ _ _ _ _ _ _ _ _ _]
      tunnel: w1109 -> [_ _ w1214 _ _ _ _ w1568 _ _ _ _ _ _ w1649 _ w1711 _ _ w2080 _ _ _ _ _ _ _ _ _ _ _ _ _ _ _ _ _ _ _ _ _ _ _ _ _]
      tunnel: w1108 -> [_ _ w1211 _ _ _ _ _ _ _ _ _ _ _ w1648 _ _ _ _ w2081 _ _ _ _ _ _ _ _ _ _ _ _ _ _ _ _ _ _ _ _ _ _ _ _ _]
      tunnel: w1107 -> [w1139 _ _ _ _ _ _ _ _ _ _ _ _ _ _ _ _ _ _ w2082 _ _ _ _ _ _ _ _ _ _ _ _ _ _ _ _ _ _ _ _ _ _ _ _ _]
      tunnel: w1106 -> [w1137 _ _ _ _ _ _ _ _ _ _ _ _ _ _ w1661 _ _ w1801 w2078 _ _ _ _ _ _ _ _ _ _ _ _ _ _ _ _ _ _ _ _ _ _ _ _ _]
      tunnel: w1105 -> [w1136 _ _ w1427 _ _ _ _ _ _ _ _ _ _ _ _ _ _ _ _ _ _ _ _ _ _ _ _ _ _ _ _ _ _ _ _ _ _ _ _ _ _ _ _ _]
      tunnel: w1104 -> [_ _ _ w1426 _ _ _ _ _ _ _ _ _ _ _ _ _ _ _ _ _ _ _ _ _ _ _ _ _ _ _ _ _ _ _ _ _ _ _ _ _ _ _ _ _]
      tunnel: w1103 -> [_ _ _ _ _ _ _ _ _ _ _ _ _ _ _ _ w1712 _ _ _ _ _ _ _ w2183 _ _ _ _ _ _ _ _ _ _ _ _ _ _ _ _ _ _ _ _]
      tunnel: w1102 -> [w1138 _ _ _ _ _ _ _ _ _ _ _ _ _ _ _ _ _ _ w2079 _ _ _ _ _ _ _ _ _ _ _ _ _ _ _ _ _ _ _ _ _ _ _ _ _]
      tunnel: w1101 -> [_ _ _ _ w1485 _ _ _ _ _ _ _ _ _ _ _ _ _ w1803 _ _ _ _ _ _ _ _ _ _ _ _ _ _ _ _ _ _ _ _ _ _ _ _ _ _]
      tunnel: w1100 -> [_ w1199 _ _ _ _ _ _ _ _ _ _ _ _ _ _ _ _ _ _ _ w2143 _ _ _ _ _ _ _ _ _ _ _ _ _ _ _ _ _ _ _ _ _ _ _]
      tunnel: w1099 -> [_ _ _ _ _ _ _ _ _ _ _ _ _ _ _ _ _ _ w1810 _ _ _ _ _ _ _ _ _ _ _ _ _ _ _ _ _ _ w2312 _ _ _ _ _ _ _]
      tunnel: w1098 -> [_ _ _ _ _ _ _ _ _ _ _ _ _ _ _ _ _ _ w1793 _ _ _ _ _ _ _ _ _ _ _ _ _ _ _ _ _ _ w2313 _ _ _ _ _ _ _]
      tunnel: w1097 -> [_ _ _ _ _ _ _ _ _ _ _ _ _ _ _ _ _ _ w1809 _ _ _ _ _ _ _ _ _ _ _ _ _ _ w2268 _ _ _ w2315 w2330 _ _ _ _ _ _]
      tunnel: w1096 -> [_ _ _ _ _ _ _ _ _ _ _ _ _ _ _ _ _ _ w1808 _ _ _ _ _ _ _ _ _ _ _ _ _ _ _ _ _ _ w2311 _ _ _ _ _ _ _]
      tunnel: "mapping freq/gamma vs T" -> [_ _ _ _ _ _ _ _ _ _ _ _ _ _ _ _ _ _ w1807 _ _ _ _ _ _ _ _ _ _ _ _ _ _ _ _ _ _ _ _ _ _ _ _ _ _]
      tunnel: w1094 -> [_ _ _ _ _ _ _ _ _ _ _ _ _ _ _ _ _ _ w1805 _ _ _ _ _ _ _ _ _ _ _ _ _ _ w2269 _ _ _ _ _ _ _ _ _ _ _]
      tunnel: w1092 -> [_ _ _ _ _ _ _ _ _ _ _ _ _ _ _ _ _ _ w1802 _ _ _ _ _ _ _ _ _ _ _ _ _ _ _ _ _ _ _ _ _ _ _ _ _ _]
      tunnel: [_ _ _ _ _ _ _ _ _ _ _ _ _ _ _ _ _ _ _ _ _ _ _ _ _ _ _ _ _ _ _ _ _ _ _ _ _ _ _ _ _ "fiter staff" _ _ _] -> _
      tunnel: w1091 -> [_ w1197 w1206 _ _ _ _ w1567 _ _ _ _ _ _ _ _ _ _ _ _ _ _ _ _ _ _ _ _ _ _ _ _ _ _ _ _ _ _ _ _ _ _ _ _ _]
      tunnel: w1090 -> [_ w1195 w1205 _ w1475 w1553 w1560 w1566 _ _ _ _ _ _ _ w1657 _ _ w1798 _ _ _ _ _ _ _ _ _ _ _ _ _ _ _ _ _ _ _ _ _ _ _ _ _ _]
      tunnel: w1089 -> [_ _ w1204 _ _ _ _ _ _ _ _ _ _ _ _ _ _ _ _ _ _ _ _ w2169 w2179 _ _ _ _ _ _ _ _ _ _ _ _ _ _ _ _ _ _ _ _]
      tunnel: w1088 -> [_ _ _ _ _ _ _ _ _ _ _ _ _ _ _ _ _ _ w1796 _ _ _ _ _ _ _ _ _ _ _ _ _ _ _ _ _ _ _ _ _ _ _ _ _ _]
      tunnel: w1087 -> [_ _ _ _ _ _ _ _ _ _ _ _ _ _ _ _ _ _ w1795 _ _ _ _ _ _ _ _ _ _ _ _ _ _ _ _ _ _ _ _ _ _ _ _ _ _]
      tunnel: w1086 -> [_ _ _ _ _ _ _ _ _ _ _ _ _ _ _ _ _ _ w1791 _ _ _ _ _ _ _ _ _ _ _ _ _ _ _ _ _ _ _ _ _ _ _ _ _ _]
      tunnel: w1085 -> [_ _ _ _ _ _ _ _ _ _ _ _ _ _ _ _ _ _ w1790 _ _ _ _ _ _ _ _ _ _ _ _ _ _ _ _ _ _ _ _ _ _ _ _ _ _]
      event "Plot: fragment": Cursor Move {
        n510 = event-data() -> ("CursIdx"=w1143:i32)  [unwired: 1 in]
        n511 = case shown="0..2, Default" w1143 {
          selector: w1143 -> [w1148 w1189]
          tunnel: w1142 -> [_ _]
          tunnel: w1141 -> [w1147 _]
          tunnel: w1140 -> [_ w1166]
          tunnel: w1139 -> [w1146 _]
          tunnel: w1138 -> [w1145 _]
          tunnel: w1137 -> [_ w1165]
          tunnel: w1136 -> [_ w1164]
          frame 0..2, Default {
            # "omega map range"
            n512 = flat-sequence {
              tunnel: w1148 -> [w1151]
              tunnel: w1146 -> [w1152]
              tunnel: [w1157] -> w1144
              tunnel: w1147 -> [w1163]
